vi "Choreo_Util_AllianceFlipRotation3d.vi"(11 "Rotation":T1={"Q_quaternion"={"R"=1.0, "V"=[0.0, 0.0, 0.0]}}) -> (3 "FlippedRotation":T1={"Q_quaternion"={"R"=1.0, "V"=[0.0, 0.0, 0.0]}})   [LabVIEW 2019, in "ChoreoLib.lvlib"]
doc: "Flips a rotation3d cluster.\n\nInputs: \n -- rotation - rotation3d - The rotation to flip.\n\nOutputs:\n -- FlippedRotation - rotation3d - The flipped cluster"
uses:
  ChoreoLib.lvlib
  <vilib>/Rock Robotics/WPI/ThirdParty/JAS_Junk/TrajLib/TypeDef/ROTATION3D.ctl
  <vilib>/Rock Robotics/WPI/ThirdParty/JAS_Junk/TrajLib/TypeDef/QUATERNION.ctl
  <vilib>/Rock Robotics/WPI/ThirdParty/JAS_Junk/TrajLib/VI/Quaternion_Get_All.vi
  <vilib>/Rock Robotics/WPI/ThirdParty/JAS_Junk/TrajLib/VI/Rotation3d_GetQuaterion.vi
  <vilib>/Rock Robotics/WPI/ThirdParty/JAS_Junk/TrajLib/Rotation2d_CreateAngle.vi
  <vilib>/Rock Robotics/WPI/ThirdParty/JAS_Junk/TrajLib/VI/Quaternion_New.vi
  <vilib>/Rock Robotics/WPI/ThirdParty/JAS_Junk/TrajLib/Rotation2d_GetAngleCosSin.vi
  <vilib>/Rock Robotics/WPI/ThirdParty/JAS_Junk/TrajLib/Rotation2d_CreateXY.vi
  <vilib>/Rock Robotics/WPI/ThirdParty/JAS_Junk/TrajLib/Util_CalcDist.vi
  Choreo_Choreo_Globals.vi
  <vilib>/Rock Robotics/WPI/ThirdParty/JAS_Junk/TrajLib/Trajectory_Library.lvlib
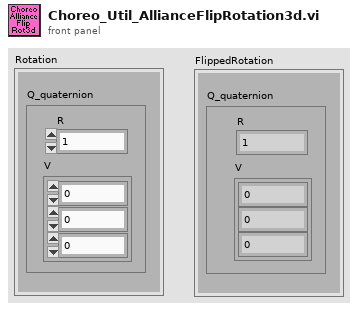
[diagram p1: front panel]
types:
  T1 = typedef "Trajectory_Library.lvlib/ROTATION3D.ctl" = cluster{"Q_quaternion":T2}
  T2 = typedef "Trajectory_Library.lvlib/QUATERNION.ctl" = cluster{"R":dbl, "V":dbl[]}
  T3 = typedef "Trajectory_Library.lvlib/ROTATION2D.ctl" = cluster{"VALUE":dbl, "COS":dbl, "SIN":dbl}
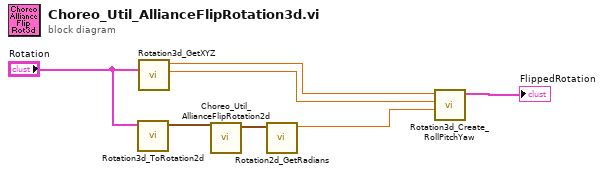
[diagram p0: block diagram]
diagram:
  n1 = call <vilib>:"Rotation3d_ToRotation2d.vi"("in Rotation3d"="Rotation") -> ("out Rotation2d"=w4:T3)  [unwired: 10 in]
  n2 = call <vilib>:"Rotation3d_GetXYZ.vi"("in Rotation3d"="Rotation") -> ("Y"=w6:dbl, "X"=w7:dbl)  [unwired: 8 in, 1 out]
  n3 = call "Choreo_Util_AllianceFlipRotation2d.vi"("Rotation"=w4) -> ("FlippedRotation"=w3:T3)  [unwired: 10 in]
  n4 = call <vilib>:"Rotation2d_GetRadians.vi"("in ROTATION"=w3) -> ("AngleRadians"=w2:dbl)  [unwired: 10 in]
  n5 = call <vilib>:"Rotation3d_Create_RollPitchYaw.vi"("Yaw"=w2, "Pitch"=w6, "Roll"=w7) -> ("Rotation3d"=→"FlippedRotation":T1)  [unwired: 8 in]
